vi "EtherNet CIP ReadBit.vi"(0 "Connection Cluster":T1={"TCP Connection"=refnum, "Session"=[], "EtherNet/IP Device Address"="172.20.37.243"} {"Session" format="0x%02x"}, 5 "Tag":string, 9 "No of Elements":u8=1, 11 "error in":errorcluster) -> (4 "Connection Cluster out":T1={"TCP Connection"=refnum, "Session"=[], "EtherNet/IP Device Address"="172.20.37.243"} {"Session" format="0x%02x"}, 6 "BOOL":bool, 15 "error out":errorcluster)   [LabVIEW 2012]
panel:
  out "Datatype":T2(ring)
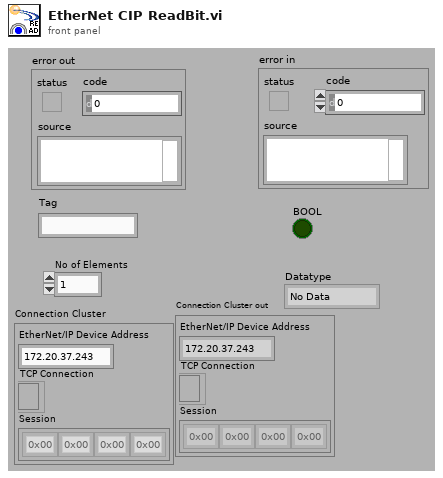
[diagram p1: front panel]
types:
  T1 = cluster{"TCP Connection":refnum<k5>, "Session":u8[], "EtherNet/IP Device Address":string}
  T2 = enum16{"No Data", "BOOL", "BIT Array", "SINT", "INT", "DINT", "REAL", "TIMER/CONTROL/COUNTER"}
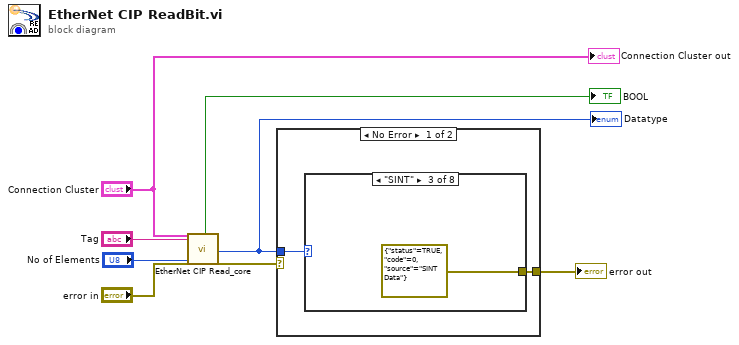
[diagram p0: block diagram]
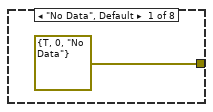
[diagram p2: hidden frame]
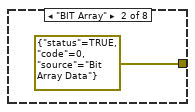
[diagram p3: hidden frame]
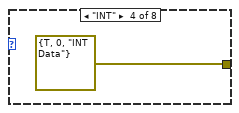
[diagram p4: hidden frame]
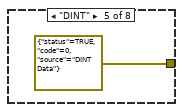
[diagram p5: hidden frame]
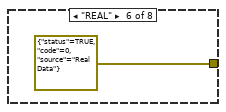
[diagram p6: hidden frame]
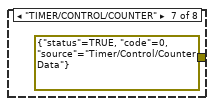
[diagram p7: hidden frame]
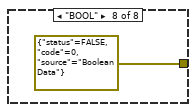
[diagram p8: hidden frame]
diagram:
  n1 = call "EtherNet CIP Read_core.vi"("Connection Cluster in"="Connection Cluster", "Tag"="Tag", "No of Elements"="No of Elements", "error in (no error)"="error in") -> ("BOOL"=→"BOOL":bool, "Datatype"=w3:T2, "error out"=w4:errorcluster)  [unwired: 14 in, 7 out]
  "Datatype" <- w3
  n2 = case shown="No Error" w4 {
    selector: w4 -> [_ w19]
    tunnel: [w10 w19] -> w8
    tunnel: w3 -> [w9 _]
    frame No Error {
      n3 = case shown="\"SINT\"" w9 {
        tunnel: [errorcluster {"status"=TRUE, "code"=0, "source"="No Data"} ("error out 2") errorcluster {"status"=TRUE, "code"=0, "source"="Bit Array Data"} ("error out 2") errorcluster {"status"=TRUE, "code"=0, "source"="SINT Data"} ("error out 2") errorcluster {"status"=TRUE, "code"=0, "source"="INT Data"} ("error out 2") errorcluster {"status"=TRUE, "code"=0, "source"="DINT Data"} ("error out 2") errorcluster {"status"=TRUE, "code"=0, "source"="Real Data"} ("error out 2") errorcluster {"status"=TRUE, "code"=0, "source"="Timer/Control/Counter Data"} ("error out 2") errorcluster {"status"=FALSE, "code"=0, "source"="Boolean Data"} ("error out 2")] -> w10
        frame "No Data", Default {
        }
        frame "BIT Array" {
        }
        frame "SINT" {
        }
        frame "INT" {
        }
        frame "DINT" {
        }
        frame "REAL" {
        }
        frame "TIMER/CONTROL/COUNTER" {
        }
        frame "BOOL" {
        }
      }
    }
    frame Error {
    }
  }
  "error out" <- w8
  "Connection Cluster out" <- "Connection Cluster"
